vi "RIOLIDARTEST.vi"() -> ()   [LabVIEW 2017]
uses:
  <vilib>/Analysis/coordinate.llb/Angle Units.ctl
  <vilib>/Analysis/coordinate.llb/Angle Range (Degree).ctl
  <vilib>/Analysis/coordinate.llb/Wrap Angle (scalar).vi
  040-typeDefs/LidarPoint.ctl
  <vilib>/gmath/NI_Gmath.lvlib
  <vilib>/ptbypt/NI_PtbyPt.lvlib
  <vilib>/Analysis/NI_AAL_Angle.lvlib
panel:
  out "Angle From WALL":dbl
  in  "y range":i32=135
  in  "y centre":i32=165
  in  "X width":i32=100
  out "Waveform Chart":cluster{"Filtered x":dbl, "Filtered x":dbl}(graph)
  out "size(s)":i32
  out "Array 2":dbl[](array[numeric])
  out "Array":cluster{dbl[], dbl[]}[](array[cluster])
  in  "stop":bool
  # "s"
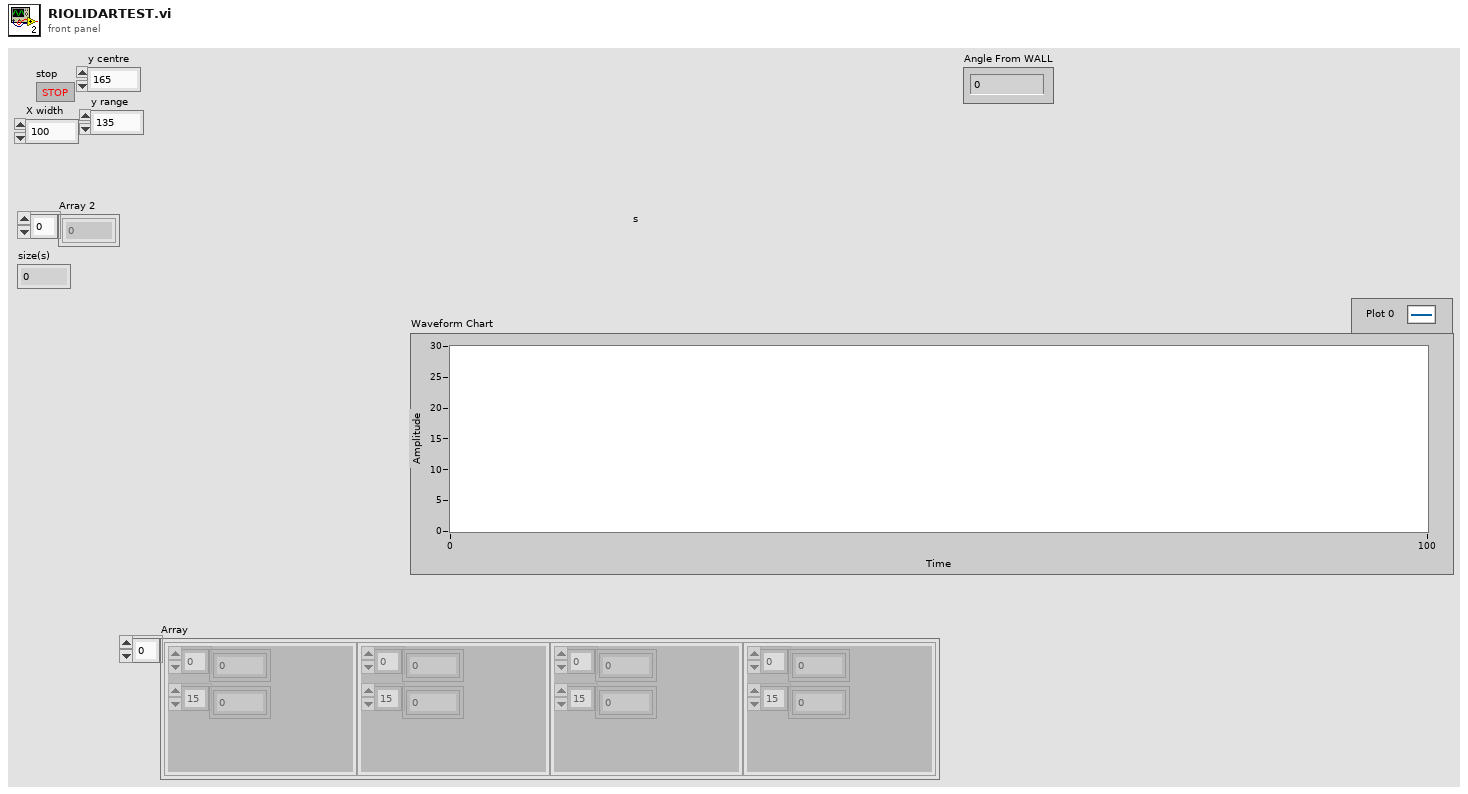
[diagram p1: front panel]
types:
  T1 = typedef "LidarPoint.ctl" = cluster{"X":dbl, "Y":dbl}
  T2 = typedef "NI_AAL_Angle.lvlib/Angle Range (Degree).ctl" = u16
  T3 = typedef "NI_AAL_Angle.lvlib/Angle Units.ctl" = i32
  T4 = typedef "XY.ctl" = T1[]
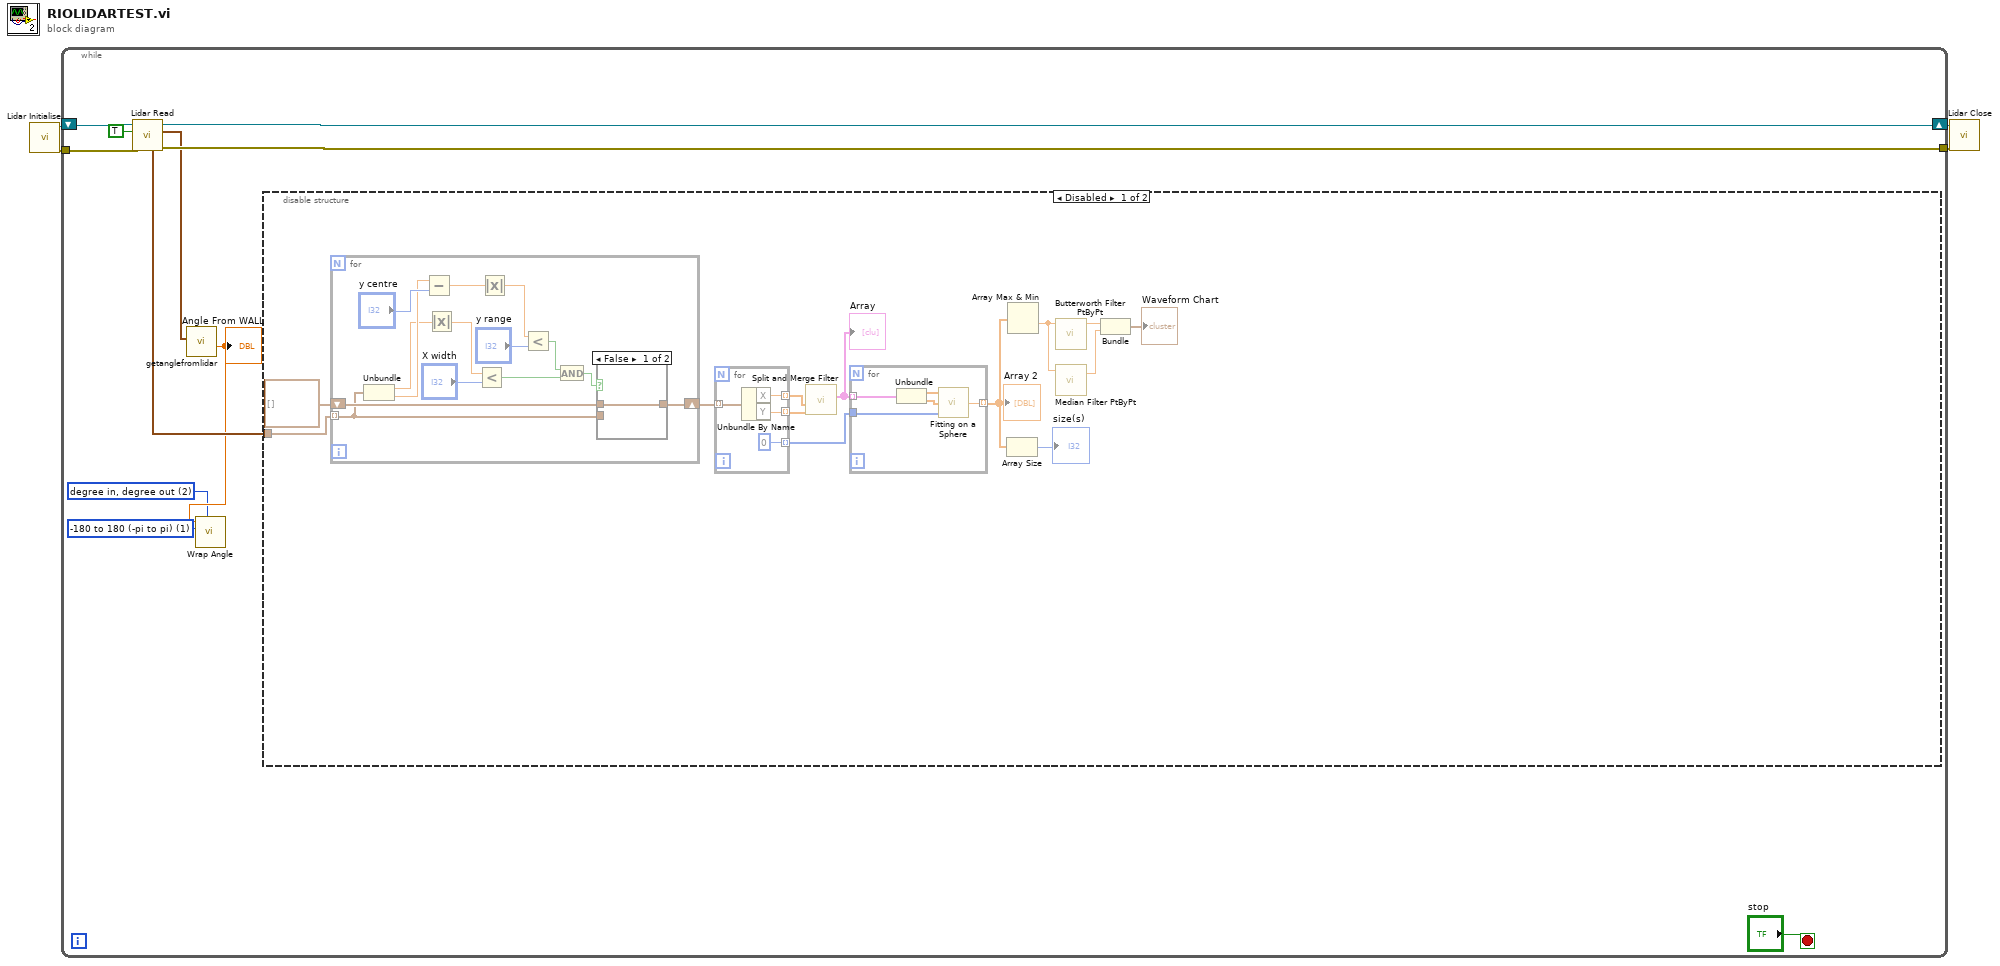
[diagram p0: block diagram]
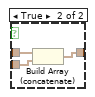
[diagram p2: hidden frame]
diagram:
  n1 = call "Lidar Initialise.vi"() -> ("error out"=w2:errorcluster, "VISA resource name out"=w4:refnum<visa-resource-name>)  [unwired: 10 in]
  n2 = while {
    shift-right: [w14] -> w3
    shift-left: w4 -> [w15]
    tunnel: w2 -> [w13]
    tunnel: [w12] -> w1
    stop <- "stop" stop-if-true
    w6 = T2 1 items=["none", "-180 to 180 (-pi to pi)", "0 to 360 (0 to 2pi)"] ("angle range")
    w7 = T3 2 items=["radian in, radian out", "radian in, degree out", "degree in, degree out", "degree in, radian out"] ("angle units")
    n3 = call "Lidar Read.vi"("error in (no error)"=w13, "Inside?"=TRUE, "VISA resource name"=w15) -> ("error out"=w12:errorcluster, "XY Array"=w9:T4, "VISA resource name out"=w14:refnum<visa-resource-name>, "Array 2"=w10:T1[])  [unwired: 3 in, 1 out]
    n4 = call "getanglefromlidar.vi"("XY Array"=w9) -> ("Angle From WALL"=w8:dbl)  [unwired: 5 in, 5 out]
    "Angle From WALL" <- w8
    n5 = call-poly <vilib>:"Wrap Angle.vi"("angle units"=w7, "angle range"=w6, "angle in"=w8) -> ()  [unwired: 7 in, 2 out]
    n6 = disable-structure shown="Disabled" {
      disable-tunnel: w10 -> [w22 _]
      frame Disabled {
        n7 = for {
          tunnel: w22 -> [w34] mode=indexing
          shift-right: [w35] -> w27
          shift-left: T1[] [] -> [w44]
          n8 = Unbundle(w34) -> ("X"=w37:dbl, "Y"=w41:dbl)
          n9 = Subtract(x=w41, y="y centre") -> (x-y=w45:dbl)
          n10 = Absolute Value(x=w37) -> (abs(x)=w38:dbl)
          n11 = Less?(x=w38, y="X width") -> (x < y?=w36:bool)
          n12 = Absolute Value(x=w45) -> (abs(x)=w46:dbl)
          n13 = Less?(x=w46, y="y range") -> (x < y?=w40:bool)
          n14 = And(x=w40, y=w36) -> (x .and. y?=w43:bool)
          n15 = case shown="False" w43 {
            tunnel: [w48 w51] -> w35
            tunnel: w44 -> [w48 w50]
            tunnel: w34 -> [_ w49]
            frame False {
            }
            frame True {
              n16 = Build Array (concatenate)(w50, w49) -> (w51:T1[])
            }
          }
        }
        n17 = for {
          tunnel: [w55] -> w25 mode=indexing
          tunnel: [w54] -> w26 mode=indexing
          tunnel: w27 -> [w53] mode=indexing
          tunnel: [0] -> w23 mode=indexing
          n18 = Unbundle By Name(w53) -> ("X"=w54:dbl, "Y"=w55:dbl)
        }
        n19 = call "Split and Merge Filter.vi"("Y"=w25, "X"=w26) -> ("Array"=w24:cluster{dbl[], dbl[]}[])  [unwired: 9 in]
        "Array" <- w24
        n20 = for {
          tunnel: w24 -> [w32] mode=indexing
          tunnel: w23 -> [w33]
          tunnel: [w29] -> w21 mode=indexing
          n21 = Unbundle(w32) -> (w31:dbl[], w30:dbl[])
          n22 = call <vilib>:"Fitting on a Sphere.vi"("Z"=w33, "Y"=w30, "X"=w31) -> ("r"=w29:dbl)  [unwired: 2 out]
        }
        "Array 2" <- w21
        n23 = Array Size(array=w21) -> (size(s)=→"size(s)":i32)
        n24 = Array Max & Min(array=w21) -> (min value=w20:dbl)  [unwired: 3 out]
        n25 = call <vilib>:"Butterworth Filter PtByPt.vi"("x"=w20) -> ("Filtered x"=w19:dbl)  [unwired: 8 in, 1 out]
        n26 = call <vilib>:"Median Filter PtByPt.vi"("x"=w20) -> ("Filtered x"=w18:dbl)  [unwired: 3 in, 1 out]
        n27 = Bundle("Filtered x"=w19, "Filtered x"=w18) -> (→"Waveform Chart":cluster{"Filtered x":dbl, "Filtered x":dbl})  [unwired: 1 in]
      }
      frame Enabled {
      }
    }
  }
  n28 = call "Lidar Close.vi"("error in (no error)"=w1, "VISA resource name"=w3) -> ()  [unwired: 9 in, 1 out]
